vi "speed test.vi"(11 "2D Color value array":T1(array[cluster])) -> ()   [LabVIEW 2015]
panel:
  out "x":dbl
  out "Numeric 2":dbl
  out "Numeric 3":dbl
  out "Array":dbl[][](array[numeric])
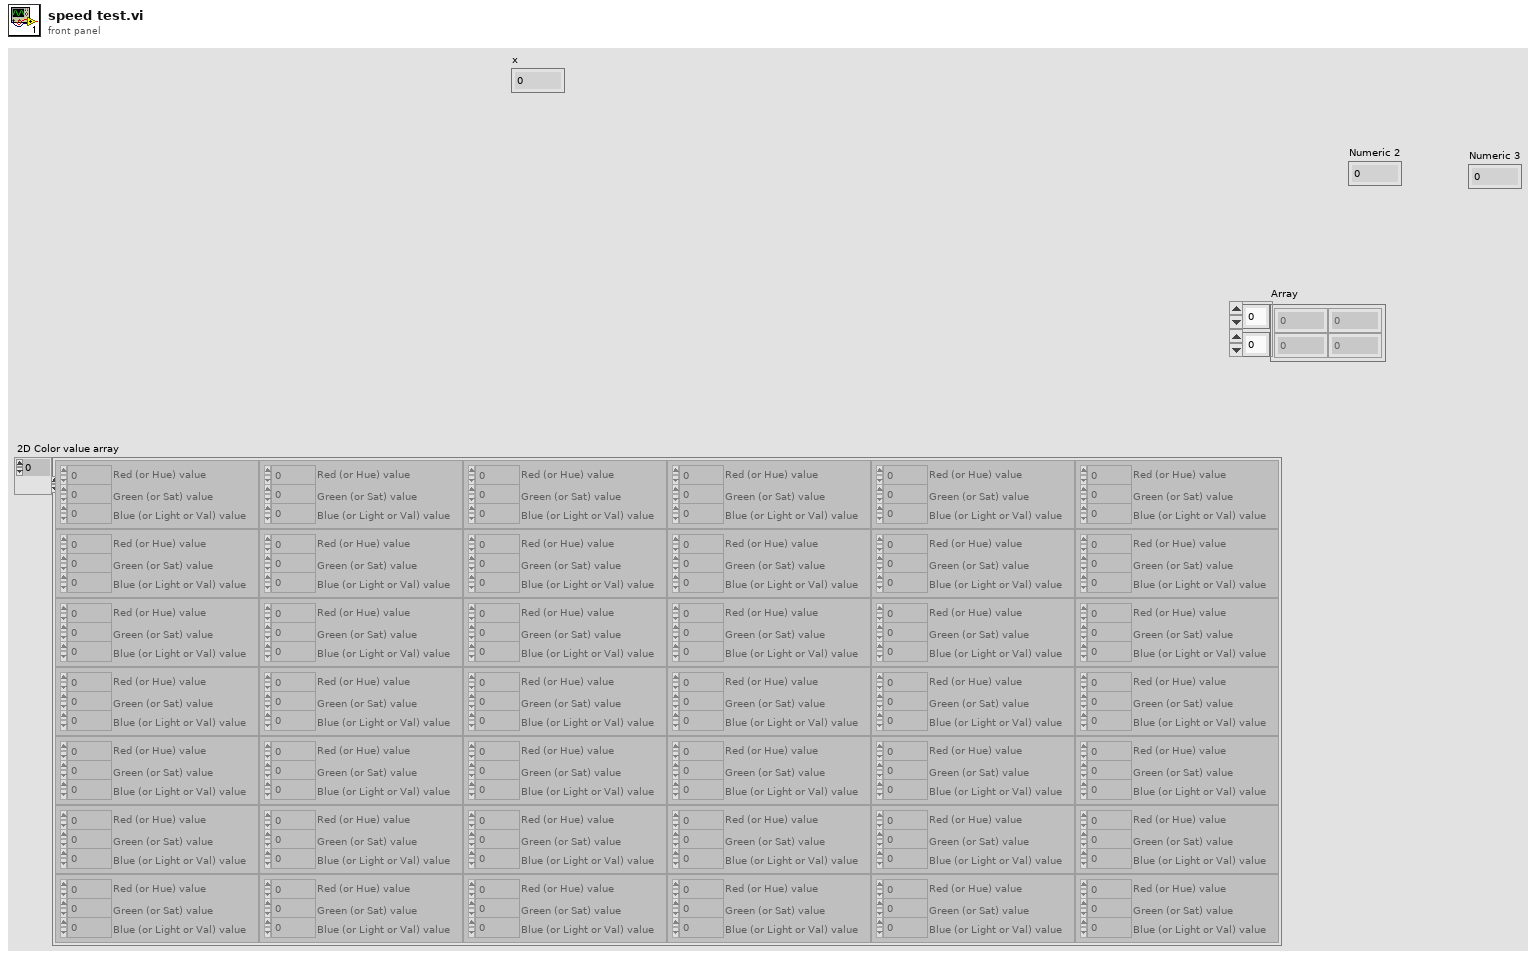
[diagram p1: front panel]
types:
  T1 = cluster{"Red (or Hue) value":u8, "Green (or Sat) value":u8, "Blue (or Light or Val) value":u8}[][]
  T2 = cluster{"Red (or Hue) value":u8, "Green (or Sat) value":u8, "Blue (or Light or Val) value":u8}
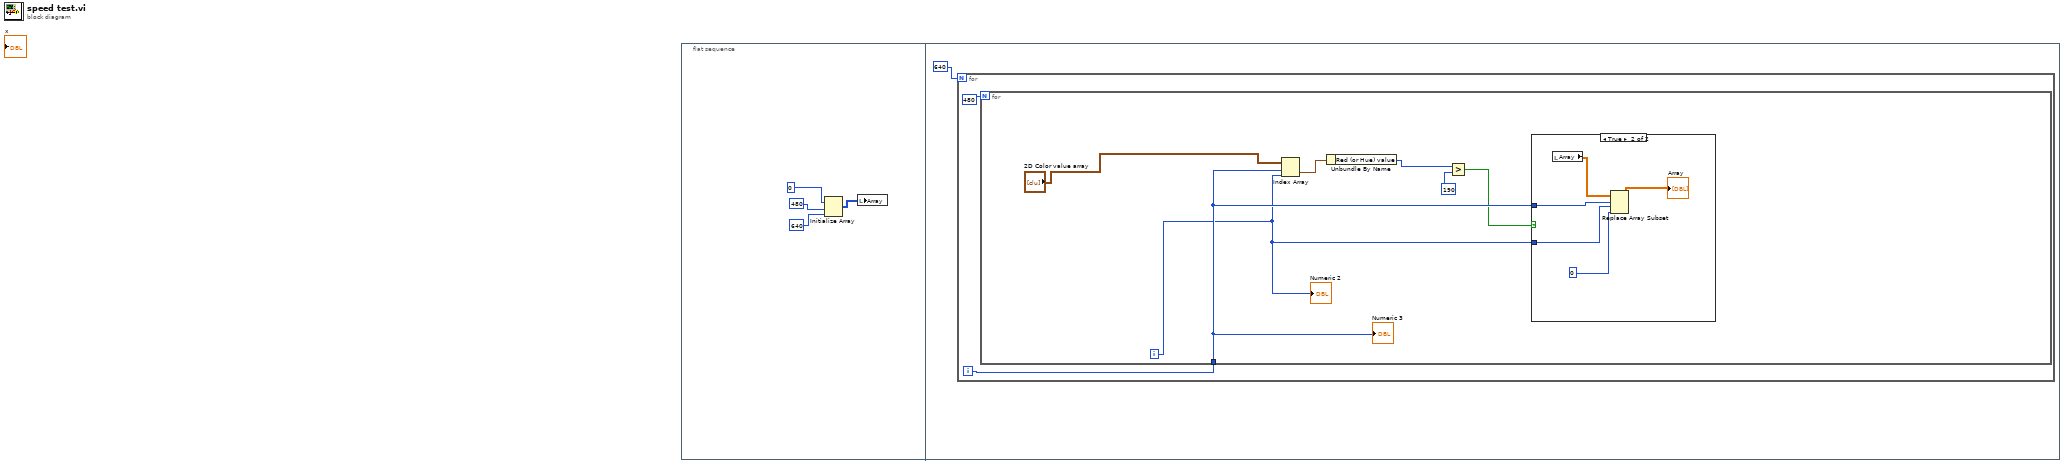
[diagram p0: block diagram]
diagram:
  n1 = flat-sequence {
    frame #0 {
      n2 = Initialize Array(0, 480, 640) -> (w1:i32[][])
      n3 = local write "Array"(w1) -> ()
    }
    frame #1 {
      n4 = for {
        N: 640 -> [_]
        i -> [w7]
        n5 = for {
          N: 480 -> [_]
          tunnel: w7 -> [w12]
          i -> [w11]
          n6 = Index Array(array="2D Color value array", index (row)=w12, index (col)=w11) -> (element=w14:T2)
          n7 = Unbundle By Name(w14) -> ("Red (or Hue) value"=w10:u8)
          n8 = Greater?(x=w10, y=190) -> (0:w9:bool)
          n9 = case shown="True" w9 {
            tunnel: w12 -> [_ w19]
            tunnel: w11 -> [_ w18]
            frame False {
            }
            frame True {
              n10 = local read "Array"() -> (w16:dbl[][])
              n11 = Replace Array Subset(array=w16, new element=0, index (row)=w19, index (col)=w18) -> (→"Array":dbl[][])
            }
          }
          "Numeric 2" <- w11
          "Numeric 3" <- w12
        }
      }
    }
  }
